vi "Cameraleg.vi"() -> ()   [LabVIEW 2018]
panel:
  out "Image Out":T1(plugin-control)
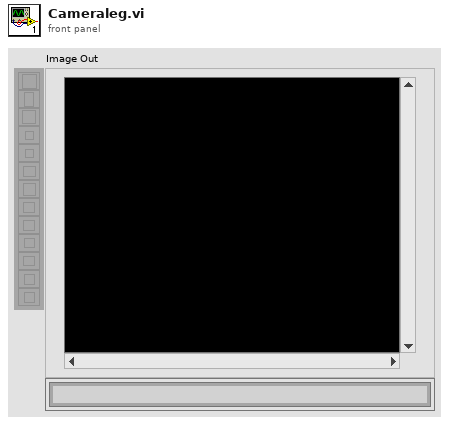
[diagram p1: front panel]
types:
  T1 = typedef "IMAQ Image.ctl" = refnum<image>
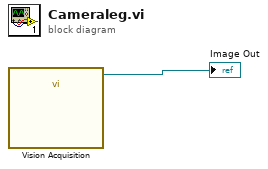
[diagram p0: block diagram]
diagram:
  n1 = call "Vision Acquisition"() -> ("Image Out"=→"Image Out":T1)  [unwired: 26 in, 1 out]
